vi "9234_UI.vi"(8 "error in (no error)":errorcluster, 11 "Node Ptr":T2 format="%.0x") -> (0 "error out":errorcluster)   [LabVIEW 2020, in "Modules.lvlib" / "9234.lvclass"]
uses:
  9234.lvclass
  <vilib>/NI VeriStand/Custom Device API/Custom Device Item Ref.ctl
  RSI Module/SubPanel Command.ctl
  Data rate.ctl
  C:/Users/nitest/Desktop/Git 2020/niveristand-scan-engine-module-libraries/Source/RSI Module/RSI Module.lvclass
  9234.lvclass/9234.ctl
  RSI Module/RSI Module.lvclass
  <vilib>/NI VeriStand/Custom Device API/Custom Device API.lvlib
panel:
  in  "ADC sampling rate":T1 items=["51.200 kS/s", "25.600 kS/s", "17.067 kS/s", "12.800 kS/s", "10.240 kS/s", "8.533 kS/s", "7.314 kS/s", "6.400 kS/s", "5.689 kS/s", "5.120 kS/s", "4.654 kS/s", "4.267 kS/s", "3.938 kS/s", "3.657 kS/s", "3.413 kS/s", "3.200 kS/s", "3.012 kS/s", "2.845 kS/s", "2.695 kS/s", "2.560 kS/s", "2.438 kS/s", "2.328 kS/s", "2.226 kS/s", "2.133 kS/s", "2.048 kS/s", "1.969 kS/s", "1.896 kS/s", "1.829 kS/s", "1.765 kS/s", "1.707 kS/s", "1.652 kS/s"]
  in  "_Input Config":u32[](array[ring]) items=["AC Coupled", "DC Coupled", "IEPE AC Coupled"]
  out "_Selected Channel(s) Settings Label":string="Selected Channel(s) Settings"
  in  "Bad Input Configuration":u8(ring) caption="Input Configuration" items=["AC Coupled", "DC Coupled", "IEPE AC Coupled", "X"]
  in  "Channels":i32[](listbox)=[0]
  in  "SubPanel Event":refnum<user-event>
  in  "Header":cluster{"Section Name":string}={"Section Name"="NI 9205 Settings"}
  in  "Input Configuration":u8(ring) items=["AC Coupled", "DC Coupled", "IEPE AC Coupled"]
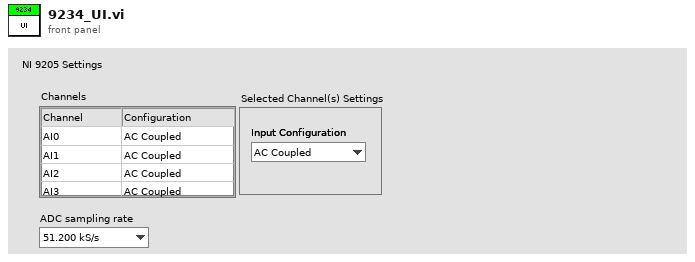
[diagram p1: front panel]
types:
  T1 = typedef "Modules.lvlib/9234.lvclass/Data rate.ctl" = u32
  T2 = typedef "Custom Device API.lvlib/Custom Device Item Ref.ctl" = u64
  T3 = typedef "Modules.lvlib/RSI Module.lvclass/Module Models.ctl" = enum16{"Empty", "NI 9201", "NI 9203", "NI 9205", "NI 9206", "NI 9207", "NI 9208", "NI 9209", "NI 9210", "NI 9211", "NI 9212", "NI 9213", "NI 9214", "NI 9215", "NI 9216", "NI 9217", "NI 9219", "NI 9220", "NI 9221", "NI 9222", "NI 9223", "NI 9224", "NI 9225", "NI 9226", "NI 9227", "NI 9228", "NI 9229", "NI 9233", "NI 9234", "NI 9235", "NI 9236", "NI 9237", "NI 9239", "NI 9242", "NI 9244", "NI 9253", "NI 9263", "NI 9264", "NI 9265", "NI 9266", "NI 9269", "NI 9344", "NI 9350", "NI 9375", "NI 9401", "NI 9402", "NI 9403", "NI 9411", "NI 9421", "NI 9422", "NI 9423", "NI 9425", "NI 9426", "NI 9435", "NI 9436", "NI 9437", "NI 9472", "NI 9474", "NI 9475", "NI 9476", "NI 9477", "NI 9478", "NI 9481", "NI 9482", "NI 9485"}
  T4 = typedef "Modules.lvlib/RSI Module.lvclass/SubPanel Command.ctl" = enum16{"Stop"}
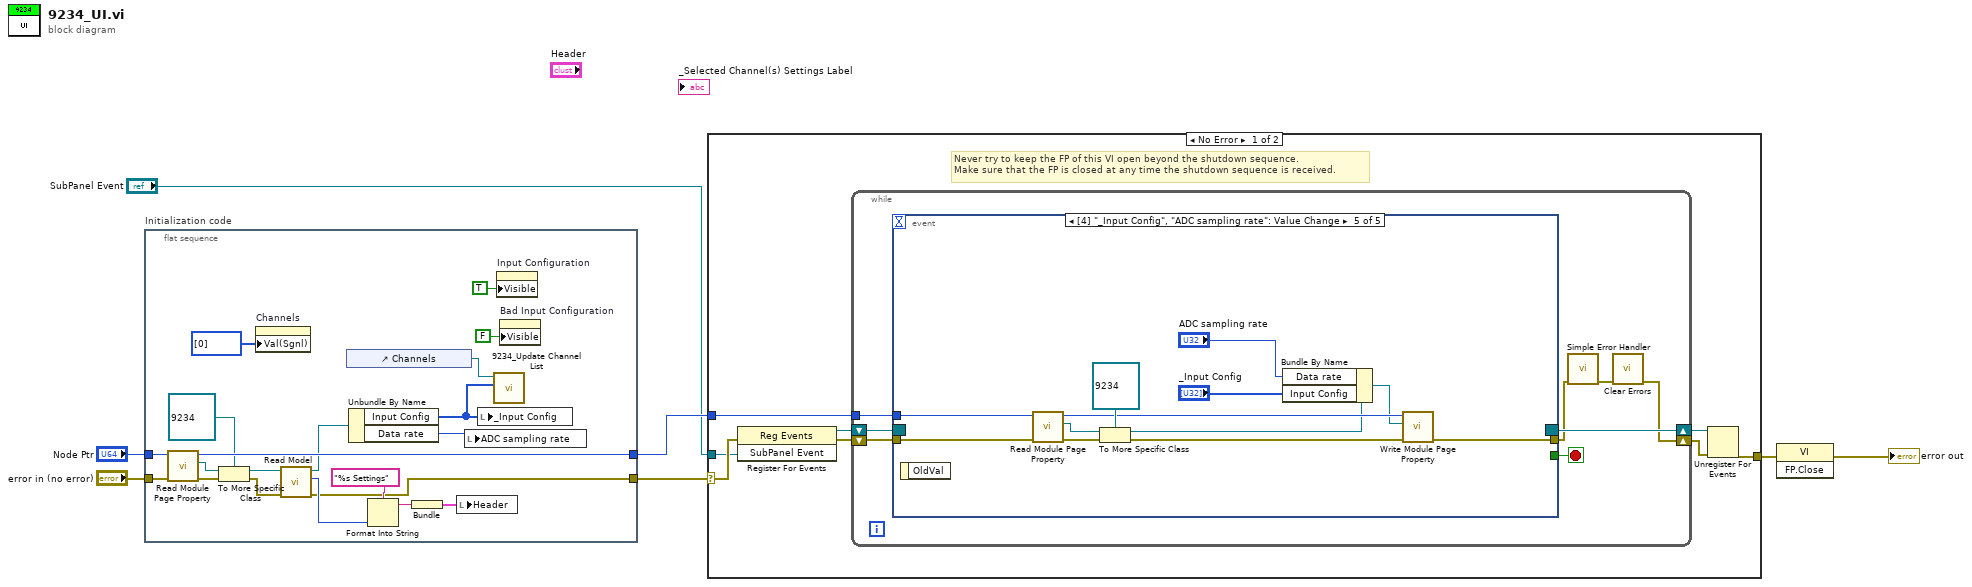
[diagram p0: block diagram]
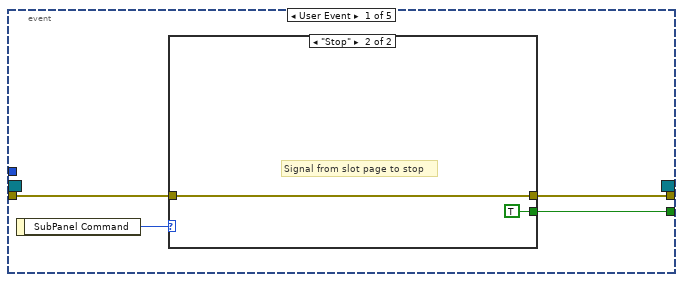
[diagram p2: hidden frame]
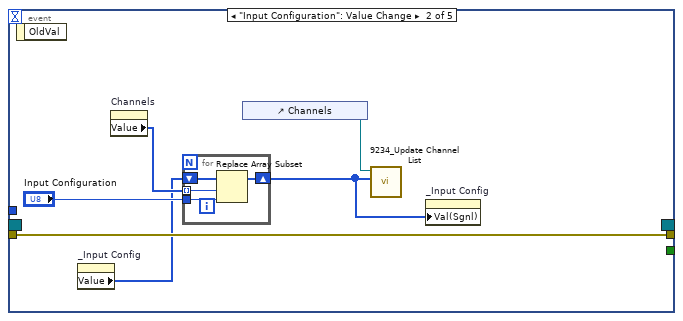
[diagram p4: hidden frame]
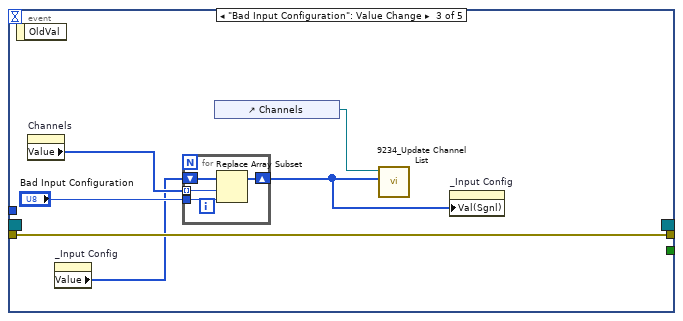
[diagram p5: hidden frame]
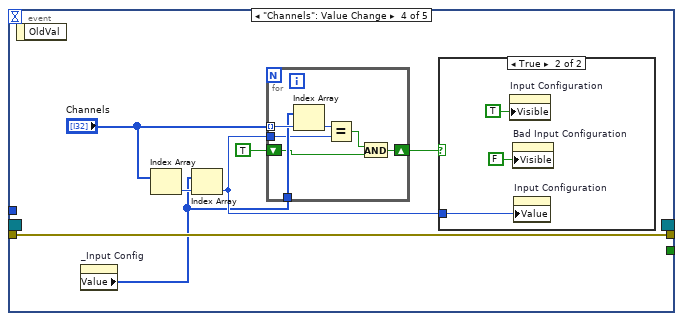
[diagram p6: hidden frame]
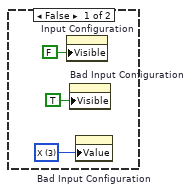
[diagram p7: hidden frame]
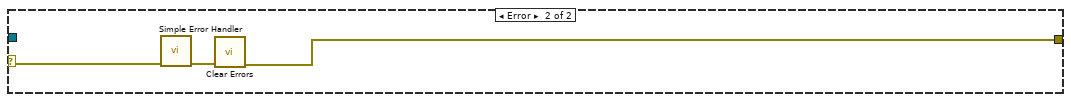
[diagram p8: hidden frame]
diagram:
  n1 = flat-sequence "Initialization code" {
    tunnel: "error in (no error)" -> [w26]
    tunnel: "Node Ptr" -> [w27]
    tunnel: [w14] -> w1
    tunnel: [w25] -> w4
    frame #0 {
      n2 = call "Read Module Page Property.vi"("error in (no error)"=w26, "Node Ptr In"=w27) -> ("error out"=w24:errorcluster, "RSI Module"=w22:refnum<class "RSI Module.lvclass">, "Node Ptr Out"=w25:T2)  [unwired: 7 in]
      n3 = To More Specific Class(target class=refnum<class "9234.lvclass"> refnum ("9205 in"), reference=w22, error in=w24) -> (specific class reference=w21:refnum<class "9234.lvclass">, error out=w20:errorcluster)
      n4 = property on="Channels" class="MCListbox (strict)"("Val(Sgnl)"=i32[] [0] ("Channels")) -> ()  [unwired: 2 in, 2 out]
      n5 = call "Read Model.vi"("error in (no error)"=w20, "RSI Module in"=w21) -> ("error out"=w14:errorcluster, "Model"=w18:T3, "RSI Module out"=w15:refnum<class "9234.lvclass">)  [unwired: 7 in]
      n6 = control-ref of="Channels"() -> (w12:refnum<vi>)
      n7 = Unbundle By Name(w15) -> ("Input Config"=w13:u32[], "Data rate"=w8:T1)
      n8 = Format Into String(format string="%s Settings", w18) -> (resulting string=w16:string)  [unwired: 2 in, 1 out]
      n9 = Bundle(w16) -> (w19:cluster{string})  [unwired: 1 in]
      n10 = local write "Header"(w19) -> ()
      n11 = local write "ADC sampling rate"(w8) -> ()
      n12 = local write "_Input Config"(w13) -> ()
      n13 = call "9234_Update Channel List.vi"("Channels"=w13, "MCListbox Refnum"=w12) -> ()  [unwired: 10 in]
      n14 = property on="Input Configuration" class="Ring (strict)"("Visible"=TRUE) -> ()  [unwired: 2 in, 2 out]
      n15 = property on="Bad Input Configuration" class="Ring (strict)"("Visible"=FALSE) -> ()  [unwired: 2 in, 2 out]
    }
  }
  n16 = case shown="No Error" w1 {
    selector: w1 -> [w29 w105]
    tunnel: [w33 w103] -> w7
    tunnel: w4 -> [w30 _]
    tunnel: "SubPanel Event" -> [w28 _]
    frame No Error {
      # "Never try to keep the FP of this VI open beyond the shutdown sequence.\nMake sure that the FP is closed at any time the shutdown sequence is received."
      n17 = register-events(error in=w29, w28) -> (reference out=w31:refnum<event-registration>, error out=w32:errorcluster)  [unwired: 1 in]
      n18 = while {
        tunnel: w30 -> [w39]
        shift-right: [w36] -> w34
        shift-left: w32 -> [w42]
        shift-right: [w43] -> w35
        shift-left: w31 -> [w41]
        stop <- w40 stop-if-true
        n19 = event shown="[4] \"_Input Config\", \"ADC sampling rate\": Value Change" {
          selector: w41 -> [_ _ _ _ _]
          dyn-events: [_ _ _ _ _] -> w43
          timeout: _ -> [_ _ _ _ _]
          tunnel: w42 -> [w46 w54 w65 w72 w96]
          tunnel: [w45 _ _ _ _] -> w40
          tunnel: [w44 w54 w65 w72 w95] -> w38
          tunnel: w39 -> [_ _ _ _ w97]
          event User Event {
            n20 = event-data() -> ("SubPanel Command"=w47:T4)  [unwired: 1 out]
            n21 = case shown="\"Stop\"" w47 {
              tunnel: w46 -> [w48 w49]
              tunnel: [w48 w49] -> w44
              tunnel: [_ TRUE] -> w45
              frame Default {
              }
              frame "Stop" {
                # "Signal from slot page to stop"
              }
            }
          }
          event "Input Configuration": Value Change {
            n22 = event-data() -> ()  [unwired: 2 out]
            n23 = property on="_Input Config" class="Arr (strict)"() -> ("Value"=w51:u32[])  [unwired: 2 in, 2 out]
            n24 = property on="Channels" class="MCListbox (strict)"() -> ("Value"=w55:i32[])  [unwired: 2 in, 2 out]
            n25 = for {
              tunnel: "Input Configuration" -> [w60]
              tunnel: w55 -> [w59] mode=indexing
              shift-right: [w57] -> w52
              shift-left: w51 -> [w58]
              n26 = Replace Array Subset(array=w58, new element=w60, index=w59) -> (w57:u32[])
            }
            n27 = control-ref of="Channels"() -> (w53:refnum<vi>)
            n28 = call "9234_Update Channel List.vi"("Channels"=w52, "MCListbox Refnum"=w53) -> ()  [unwired: 10 in]
            n29 = property on="_Input Config" class="Arr (strict)"("Val(Sgnl)"=w52) -> ()  [unwired: 2 in, 2 out]
          }
          event "Bad Input Configuration": Value Change {
            n30 = event-data() -> ()  [unwired: 2 out]
            n31 = property on="Channels" class="MCListbox (strict)"() -> ("Value"=w66:i32[])  [unwired: 2 in, 2 out]
            n32 = property on="_Input Config" class="Arr (strict)"() -> ("Value"=w61:u32[])  [unwired: 2 in, 2 out]
            n33 = for {
              tunnel: "Bad Input Configuration" -> [w70]
              tunnel: w66 -> [w69] mode=indexing
              shift-right: [w67] -> w62
              shift-left: w61 -> [w68]
              n34 = Replace Array Subset(array=w68, new element=w70, index=w69) -> (w67:u32[])
            }
            n35 = control-ref of="Channels"() -> (w63:refnum<vi>)
            n36 = call "9234_Update Channel List.vi"("Channels"=w62, "MCListbox Refnum"=w63) -> ()  [unwired: 10 in]
            n37 = property on="_Input Config" class="Arr (strict)"("Val(Sgnl)"=w62) -> ()  [unwired: 2 in, 2 out]
          }
          event "Channels": Value Change {
            n38 = event-data() -> ()  [unwired: 2 out]
            n39 = property on="_Input Config" class="Arr (strict)"() -> ("Value"=w71:u32[])  [unwired: 2 in, 2 out]
            n40 = Index Array(array="Channels") -> (element=w77:i32)  [unwired: 1 in]
            n41 = Index Array(array=w71, index=w77) -> (element=w73:u32)
            n42 = for {
              tunnel: "Channels" -> [w89] mode=indexing
              tunnel: w71 -> [w88]
              tunnel: w73 -> [w86]
              shift-right: [w84] -> w74
              shift-left: TRUE -> [w85]
              n43 = Index Array(array=w88, index=w89) -> (element=w87:u32)
              n44 = Equal?(x=w87, y=w86) -> (x = y?=w90:bool)
              n45 = And(x=w90, y=w85) -> (x .and. y?=w84:bool)
            }
            n46 = case shown="True" w74 {
              tunnel: w73 -> [_ w81]
              frame False {
                w78 = u8 3 items=["AC Coupled", "DC Coupled", "IEPE AC Coupled", "X"]
                n47 = property on="Input Configuration" class="Ring (strict)"("Visible"=FALSE) -> ()  [unwired: 2 in, 2 out]
                n48 = property on="Bad Input Configuration" class="Ring (strict)"("Visible"=TRUE) -> ()  [unwired: 2 in, 2 out]
                n49 = property on="Bad Input Configuration" class="Ring (strict)"("Value"=w78) -> ()  [unwired: 2 in, 2 out]
              }
              frame True {
                n50 = property on="Input Configuration" class="Ring (strict)"("Visible"=TRUE) -> ()  [unwired: 2 in, 2 out]
                n51 = property on="Bad Input Configuration" class="Ring (strict)"("Visible"=FALSE) -> ()  [unwired: 2 in, 2 out]
                n52 = property on="Input Configuration" class="Ring (strict)"("Value"=w81) -> ()  [unwired: 2 in, 2 out]
              }
            }
          }
          event "_Input Config": Value Change {
            n53 = event-data() -> ()  [unwired: 2 out]
            n54 = call "Read Module Page Property.vi"("error in (no error)"=w96, "Node Ptr In"=w97) -> ("error out"=w100:errorcluster, "RSI Module"=w101:refnum<class "RSI Module.lvclass">, "Node Ptr Out"=w98:T2)  [unwired: 7 in]
            n55 = To More Specific Class(target class=refnum<class "9234.lvclass"> refnum ("9205 in"), reference=w101, error in=w100) -> (specific class reference=w94:refnum<class "9234.lvclass">, error out=w99:errorcluster)
            n56 = Bundle By Name(cluster=w94, "Data rate"="ADC sampling rate", "Input Config"="_Input Config") -> (w93:refnum<class "9234.lvclass">)
            n57 = call "Write Module Page Property.vi"("error in (no error)"=w99, "RSI Module"=w93, "Node Ptr In"=w98) -> ("error out"=w95:errorcluster)  [unwired: 6 in, 2 out]
          }
        }
        n58 = call <vilib>:"Simple Error Handler.vi"("error in (no error)"=w38) -> ("error out"=w37:errorcluster)  [unwired: 1 in, 7 out]
        n59 = call <vilib>:"Clear Errors.vi"("error in (no error)"=w37) -> ("error out"=w36:errorcluster)  [unwired: 1 in, 5 out]
      }
      n60 = Unregister For Events(event registration refnum=w35, error in=w34) -> (error out=w33:errorcluster)
    }
    frame Error {
      n61 = call <vilib>:"Simple Error Handler.vi"("error in (no error)"=w105) -> ("error out"=w104:errorcluster)  [unwired: 1 in, 7 out]
      n62 = call <vilib>:"Clear Errors.vi"("error in (no error)"=w104) -> ("error out"=w103:errorcluster)  [unwired: 1 in, 5 out]
    }
  }
  n63 = invoke class="VI" method="FP.Close"(error in=w7) -> (error out=→"error out":errorcluster)  [unwired: 2 in, 2 out]
